vi "定位数据源.vi"(8 "错误输入（无错误）":errorcluster) -> (0 "错误输出":errorcluster, 3 "数据":refnum<k7>)   [LabVIEW 2011]
panel:
  in  "ADODB._Connection":refnum<k7>
  in  "MSDASC.IDataSourceLocator":refnum<k7>
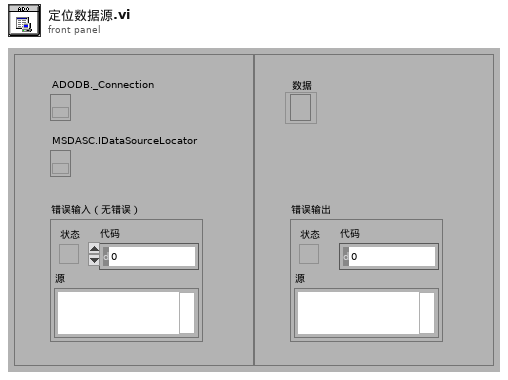
[diagram p1: front panel]
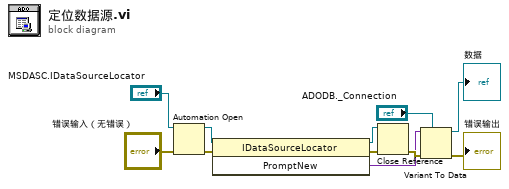
[diagram p0: block diagram]
diagram:
  n1 = Automation Open(error in (no error)="错误输入（无错误）", Automation Refnum="MSDASC.IDataSourceLocator") -> (Automation Refnum=w11:refnum<k7>, error out=w9:errorcluster)  [unwired: 2 out]
  n2 = invoke class="IDataSourceLocator" method="PromptNew"(reference=w11, error in=w9) -> (reference out=w5:refnum<k7>, error out=w6:errorcluster, "PromptNew"=w7:variant)  [unwired: 1 in]
  n3 = Close Reference(reference=w5, error in (no error)=w6) -> (error out=w8:errorcluster)
  n4 = Variant To Data(error in=w8, type="ADODB._Connection", Variant=w7) -> (data=→"数据":refnum<k7>, error out=→"错误输出":errorcluster)
